vi "Channel List String.vi"(9 "Enable Channel 1 to 2":bool, 10 "Channel List ({Channel1})":i32[](array[ring])=[0] items=["Channel 1", "Channel 2"]) -> (2 "Channel List Command String":string)   [LabVIEW 2020, in "Agilent B2900 Series.lvlib"]
doc: "Parse the channel list to SCPI cmd string."
uses:
  Agilent B2900 Series.lvlib
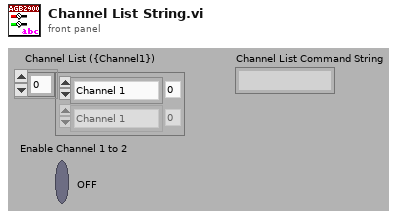
[diagram p1: front panel]
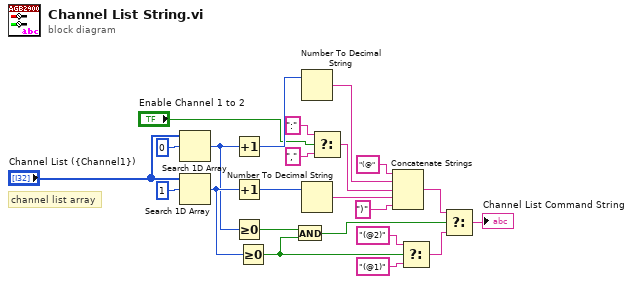
[diagram p0: block diagram]
diagram:
  # "channel list array"
  n1 = Search 1D Array(1D array="Channel List ({Channel1})", element=0) -> (index of element=w9:i32)  [unwired: 1 in]
  n2 = Search 1D Array(1D array="Channel List ({Channel1})", element=1) -> (index of element=w11:i32)  [unwired: 1 in]
  n3 = Increment(x=w9) -> (x+1=w8:i32)
  n4 = Increment(x=w11) -> (x+1=w10:i32)
  n5 = Greater Or Equal To 0?(x=w9) -> (x >= 0?=w20:bool)
  n6 = Greater Or Equal To 0?(x=w11) -> (x >= 0?=w18:bool)
  n7 = And(x=w20, y=w18) -> (x .and. y?=w19:bool)
  n8 = Number To Decimal String(number=w8) -> (decimal integer string=w5:string)  [unwired: 1 in]
  n9 = Number To Decimal String(number=w10) -> (decimal integer string=w4:string)  [unwired: 1 in]
  n10 = Select(t=":", s="Enable Channel 1 to 2", f=",") -> (s? t:f=w7:string)
  n11 = Concatenate Strings("(@", w5, w7, w4, ")") -> (w2:string)
  n12 = Select(t="(@2)", s=w18, f="(@1)") -> (s? t:f=w15:string)
  n13 = Select(t=w2, s=w19, f=w15) -> (s? t:f=→"Channel List Command String":string)
